vi "Execute Nested Msg.vi"(6 "Timeout(-1ms)":i32=-1, 7 "Response Data Type":refnum<class "Data.lvclass">, 8 "error in (no error)":errorcluster, 9 "Instrument Msg to Run":refnum<class "Instrument Msg.lvclass">, 10 "Actor in":refnum<class "Actor.lvclass">, 11 "Multi Instrument Msg in":refnum<class "Multi Instrument Msg.lvclass">) -> (0 "error out":errorcluster, 1 "Data":refnum<class "Data.lvclass">, 2 "Actor out":refnum<class "Actor.lvclass">, 3 "Multi Instrument Msg out":refnum<class "Multi Instrument Msg.lvclass">, 5 "Success?":bool)   [LabVIEW 2020, in "Instrument Handler.lvlib" / "Multi Instrument Msg.lvclass"]
doc: "Execute an Instrument Msg from the Multi Instrument Msg. Multi Instrument Msgs are also supported. \nThe returned data is casted using Preserve Run-Time Class. If the cast fails due to the wiring of an incorrect Data class success will be set to FALSE even if the instrument message executed successfully."
uses:
  Multi Instrument Msg.lvclass
  C:/Current projects/WS/Framework/Framework/Actors/Instrument Handler/Messages/Instrument Msg/Instrument Msg.lvclass
  C:/Current projects/WS/PPL/HDH.Actor Framework.Core.Msg.lvlibp/Flex Msg/Flex Msg.lvclass
  Instrument Msg/Instrument Msg.lvclass
  C:/Current projects/WS/PPL/HDH.Actor Framework.Core.Publisher.lvlibp/Messages/Response Msg/Response Msg.lvclass
  PPL/HDH.Actor Framework.Core.Actor.lvlibp/1abvi3w/vi.lib/ActorFramework/Actor/Actor.lvclass
  PPL/HDH.Data.Generic.lvlibp/Data.lvclass
  Multi Instrument Msg.lvclass/Multi Instrument Msg.ctl
  PPL/HDH.Actor Framework.Core.Sequencer.lvlibp/Sequencer Core/Sequencer Core.lvclass
  PPL/HDH.Actor Framework.Core.Publisher.lvlibp/Messages/Response Msg/Response Core/Controls/Ctl_SendFunction.ctl
  PPL/HDH.Actor Framework.Core.Actor.lvlibp/1abvi3w/vi.lib/ActorFramework/Message Enqueuer/Message Priority.ctl
  Instrument Sequencer Sender Msg/Instrument Sequencer Sender Msg.lvclass/Instrument Sequencer Sender Msg.ctl
  Instrument Sequencer Sender Msg/Instrument Sequencer Sender Msg.lvclass
  C:/Current projects/WS/PPL/HDH.Actor Framework.Core.Publisher.lvlibp/Publisher Messages/Sender Msg/Sender Msg.lvclass
  PPL/HDH.Data.Generic.lvlibp
  PPL/HDH.Actor Framework.Core.Publisher.lvlibp/Messages/Response Msg/Response Msg.lvclass
  PPL/HDH.Actor Framework.Core.Publisher.lvlibp
  PPL/HDH.Actor Framework.Core.Actor.lvlibp/1abvi3w/vi.lib/ActorFramework/Message Enqueuer/Message Enqueuer.lvclass
  PPL/HDH.Actor Framework.Core.Instrument Driver.lvlibp/Instrument Driver/Instrument Driver.lvclass
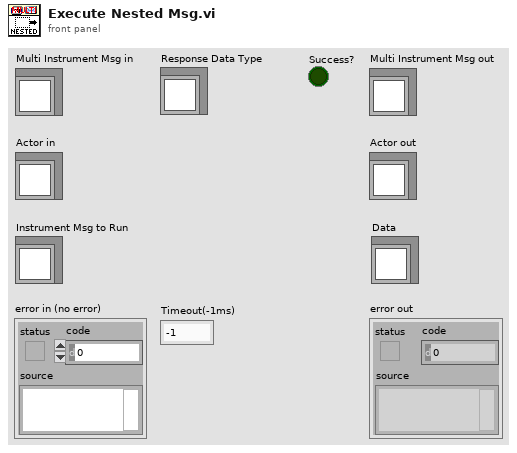
[diagram p1: front panel]
types:
  T1 = typedef "HDH.Actor Framework.Core.Actor.lvlibp/Message Enqueuer.lvclass/Message Priority.ctl" = enum16{"Low", "Normal", "High"}
  T2 = typedef "HDH.Actor Framework.Core.Publisher.lvlibp/Ctl_SendFunction.ctl" = enum16{"Send and Forget", "Request Reply", "Await Reply"}
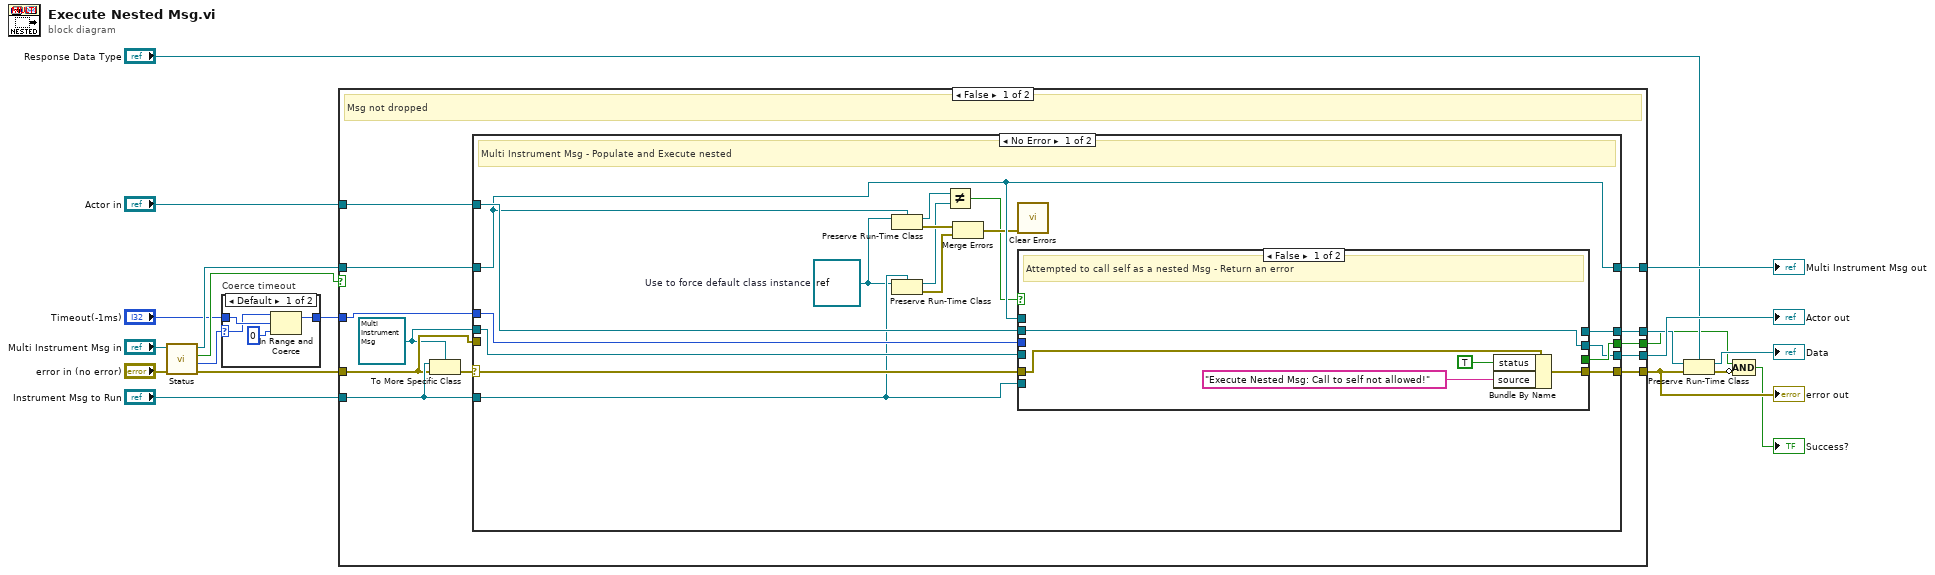
[diagram p0: block diagram]
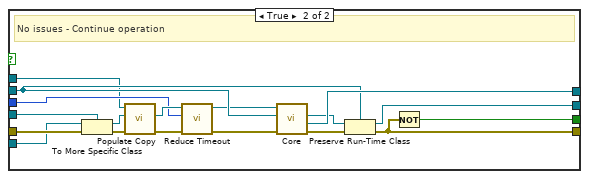
[diagram p3: hidden frame]
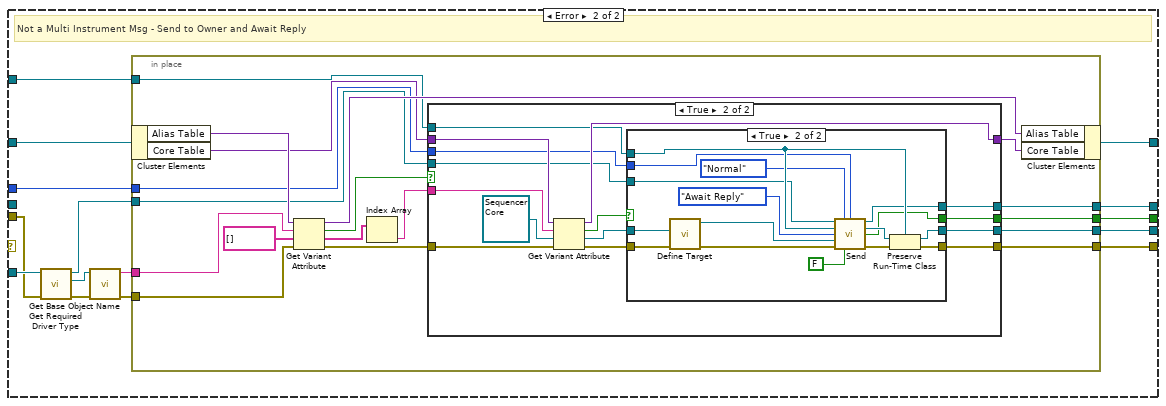
[diagram p4: hidden frame]
diagram:
  n1 = call "Status.vi"("error in (no error)"="error in (no error)", "Response Msg in"="Multi Instrument Msg in") -> ("error out"=w12:errorcluster, "Time to Timeout (ms)"=w10:i32, "Dropped?"=w11:bool, "Response Msg out"=w13:refnum<class "Multi Instrument Msg.lvclass">)  [unwired: 6 in]
  n2 = case "Coerce timeout" shown="Default" w10 {
    selector: w10 -> [w21 _]
    tunnel: [w20 w24] -> w8
    tunnel: "Timeout(-1ms)" -> [w23 w24]
    frame Default {
      n3 = In Range and Coerce(upper limit=w21, x=w23, lower limit=0) -> (coerced(x)=w20:i32)  [unwired: 1 out]
    }
    frame -1 {
    }
  }
  n4 = case shown="False" w11 {
    tunnel: [w33 w146] -> w4
    tunnel: [w29 w148] -> w19
    tunnel: w13 -> [w36 w148]
    tunnel: "Instrument Msg to Run" -> [w35 _]
    tunnel: [w31 w147] -> w17
    tunnel: "Actor in" -> [w32 w147]
    tunnel: w8 -> [w30 _]
    tunnel: [w28 _] -> w6
    tunnel: [w27 _] -> w3
    tunnel: w12 -> [w26 w146]
    frame False {
      w25 = refnum<class "Multi Instrument Msg.lvclass"> refnum ("Multi Instrument Msg in")
      # "Msg not dropped"
      n5 = To More Specific Class(target class=w25, reference=w35, error in=w26) -> (error out=w34:errorcluster)  [unwired: 1 out]
      n6 = case shown="No Error" w34 {
        selector: w34 -> [w52 _]
        tunnel: w36 -> [w45 w89]
        tunnel: w35 -> [w44 w86]
        tunnel: w26 -> [_ w85]
        tunnel: [w47 w84] -> w33
        tunnel: w32 -> [w48 w83]
        tunnel: [w49 w82] -> w31
        tunnel: w30 -> [w46 w81]
        tunnel: [w45 w79] -> w29
        tunnel: [w51 w78] -> w28
        tunnel: [w50 w77] -> w27
        tunnel: w25 -> [w53 _]
        frame No Error {
          w43 = refnum<class> refnum  # Use to force default class instance
          # "Multi Instrument Msg - Populate and Execute nested"
          n7 = Preserve Run-Time Class(object in=w43, 2:w45) -> (object out=w39:refnum<class "Multi Instrument Msg.lvclass">, error out=w42:errorcluster)  [unwired: 1 in]
          n8 = Preserve Run-Time Class(object in=w43, 2:w44) -> (object out=w38:refnum<class "Instrument Msg.lvclass">, error out=w41:errorcluster)  [unwired: 1 in]
          n9 = Not Equal?(x=w39, y=w38) -> (x != y?=w37:bool)
          n10 = Merge Errors(w42, w41) -> (w40:errorcluster)
          n11 = call <vilib>:"Clear Errors.vi"("error in (no error)"=w40) -> ()  [unwired: 5 in, 2 out]
          n12 = case shown="False" w37 {
            tunnel: w53 -> [_ w76]
            tunnel: w52 -> [w57 w75]
            tunnel: [_ w74] -> w51
            tunnel: [_ w73] -> w50
            tunnel: [w58 w71] -> w49
            tunnel: w48 -> [w58 w70]
            tunnel: [w54 w68] -> w47
            tunnel: w46 -> [_ w63]
            tunnel: w45 -> [_ w60]
            tunnel: w44 -> [_ w59]
            frame False {
              # "Attempted to call self as a nested Msg - Return an error"
              n13 = Bundle By Name(cluster=w57, "status"=TRUE, "source"="Execute Nested Msg: Call to self not allowed!") -> (w54:errorcluster)
            }
            frame True {
              # "No issues - Continue operation"
              n14 = To More Specific Class(target class=w76, reference=w59, error in=w75) -> (specific class reference=w67:refnum<class "Multi Instrument Msg.lvclass">, error out=w66:errorcluster)
              n15 = call-dynamic "Populate Copy.vi"("error in (no error)"=w66, "Msg to Populate"=w67, "Source Msg"=w60) -> ("error out"=w62:errorcluster, "Populated Msg"=w65:refnum<class "Multi Instrument Msg.lvclass">)  [unwired: 7 in]
              n16 = call "Reduce Timeout.vi"("error in (no error)"=w62, "New Timeout time(ms)"=w63, "Response Msg in"=w65) -> ("error out"=w61:errorcluster, "Response Msg out"=w64:refnum<class "Multi Instrument Msg.lvclass">)  [unwired: 6 in, 1 out]
              n17 = call-dynamic "Core.vi"("error in (no error)"=w61, "Actor in"=w70, "Multi Instrument Msg in"=w64) -> ("error out"=w69:errorcluster, "Data"=w74:refnum<class "Data.lvclass">, "Actor out"=w72:refnum<class "Actor.lvclass">)  [unwired: 5 in, 1 out]
              n18 = Preserve Run-Time Class(object in=w72, error in=w69, 2:w70) -> (object out=w71:refnum<class "Actor.lvclass">, error out=w68:errorcluster)
              n19 = Not(x=w68) -> (.not. x?=w73:bool)
            }
          }
        }
        frame Error {
          # "Not a Multi Instrument Msg - Send to Owner and Await Reply"
          n20 = call-dynamic "Get Required Driver Type.vi"("error in (no error)"=w85, "Instrument Msg in"=w86) -> ("error out"=w90:errorcluster, "Required Driver Type"=w91:refnum<class "Instrument Driver.lvclass">, "Instrument Msg out"=w80:refnum<class "Instrument Msg.lvclass">)  [unwired: 7 in]
          n21 = call "Get Base Object Name.vi"("error in (no error)"=w90, "Object in"=w91) -> ("error out"=w87:errorcluster, "Base class name"=w88:string)  [unwired: 8 in]
          n22 = in-place {
            in-place-border: w88 -> [w105]
            in-place-border: w87 -> [w104]
            in-place-border: [w98] -> w84
            in-place-border: w83 -> [w97]
            in-place-border: [w96] -> w82
            in-place-border: w81 -> [w95]
            in-place-border: w80 -> [w94]
            in-place-border: [w93] -> w78
            in-place-border: [w92] -> w77
            n23 = in-place-cluster #1(w89) -> ("Alias Table"=w107:variant, "Core Table"=w101:variant)
            n24 = Get Variant Attribute(Variant=w107, name=w105, default value (empty Variant)=string[] [] ("Base class name"), error in=w104) -> (duplicate Variant=w106:variant, found=w103:bool, value=w108:string[], error out=w99:errorcluster)
            n25 = Index Array(array=w108) -> (element=w100:string)  [unwired: 1 in]
            n26 = case shown="True" w103 {
              tunnel: [w112 w126] -> w102
              tunnel: w101 -> [w112 w127]
              tunnel: w100 -> [_ w125]
              tunnel: w99 -> [w111 w124]
              tunnel: [w111 w120] -> w98
              tunnel: w97 -> [w110 w118]
              tunnel: [w110 w117] -> w96
              tunnel: w95 -> [_ w116]
              tunnel: w94 -> [_ w115]
              tunnel: [_ w114] -> w93
              tunnel: [_ w113] -> w92
              frame False {
              }
              frame True {
                n27 = Get Variant Attribute(Variant=w127, name=w125, default value (empty Variant)=refnum<class "Sequencer Core.lvclass"> refnum ("HDH.Actor Framework.Core.Sequencer.lvlibp:Sequencer Core.lvclass"), error in=w124) -> (duplicate Variant=w126:variant, found=w122:bool, value=w121:refnum<class "Sequencer Core.lvclass">, error out=w119:errorcluster)
                n28 = case shown="True" w122 {
                  tunnel: w121 -> [_ w145]
                  tunnel: [w129 w130] -> w120
                  tunnel: w119 -> [w129 w144]
                  tunnel: w118 -> [w128 w138]
                  tunnel: [w128 w139] -> w117
                  tunnel: w116 -> [_ w136]
                  tunnel: w115 -> [_ w134]
                  tunnel: [_ w133] -> w114
                  tunnel: [_ w132] -> w113
                  frame False {
                  }
                  frame True {
                    n29 = call "Define Target.vi"("error in (no error)"=w144, "Core"=w145) -> ("error out"=w142:errorcluster, "Instrument Sequencer Sender out"=w143:refnum<class "Instrument Sequencer Sender Msg.lvclass">)  [unwired: 8 in]
                    n30 = call "Send.vi"("Response Msg in"=w134, "Message Priority (Normal)"=Message_Priority."Normal", "Timeout if waiting(-1ms)"=w136, "Actor in"=w138, "Send Function"=Ctl_SendFunction."Await Reply", "Sender (publish)"=w143, "error in (no error)"=w142, "Publish Data?(F)"=FALSE) -> ("Data"=w133:refnum<class "Data.lvclass">, "Actor out"=w140:refnum<class "Actor.lvclass">, "Success?"=w132:bool, "error out"=w131:errorcluster)  [unwired: 3 in, 1 out]
                    n31 = Preserve Run-Time Class(object in=w140, error in=w131, 2:w138) -> (object out=w139:refnum<class "Actor.lvclass">, error out=w130:errorcluster)
                  }
                }
              }
            }
            n32 = in-place-cluster #1("Alias Table"=w106, "Core Table"=w102) -> (w79:refnum<class "Multi Instrument Msg.lvclass">)
          }
        }
      }
    }
    frame True {
      # "Msg dropped"
    }
  }
  "error out" <- w4
  "Multi Instrument Msg out" <- w19
  "Actor out" <- w17
  n33 = Preserve Run-Time Class(object in=w6, error in=w4, 2:"Response Data Type") -> (object out=→"Data":refnum<class "Data.lvclass">, error out=w2:errorcluster)
  n34 = Compound Arithmetic op=AND(w3, invert w2) -> (→"Success?":bool)
